vi "Calculate Velocity Setpoints.vi"(0 "Negated":bool, 1 "Front is Back":bool, 3 "Reversed":bool, 4 "Iterations":i32, 5 "Time":u32, 6 "Velocity Data":dbl[](array[numeric]), 7 "Angular Data (Relative)":dbl[](array[numeric]), 9 "Align?":bool, 11 "Enum":enum16{"Vantage", "Mule", "Linda/Sophie"}(ring), 12 "Angle To Get":dbl(slide) scale=0.0..360.0, 13 "IMU Input":dbl, 17 "Commands":cluster{"Time (s)":dbl, T1, bool}[](array[cluster])) -> (2 "Angles PID M":cluster{"Numeric":dbl, "IMU Input":dbl}(graph), 14 "Left Setpoint":dbl, 15 "Wait Time (ms)":dbl, 18 "Finished?":bool, 19 "Right Setpoint":dbl)   [LabVIEW 2019]
uses:
  Bordeaux/Command Stuff/Single Cmd Info.ctl
  <vilib>/picture/picture.llb/imagedata.ctl
  <vilib>/addons/control/pid/pid.llb/PID (DBL).vi
  2020 Robot/Framework/Robot Global Data.vi
  <vilib>/addons/control/pid/NI_PID_pid.lvlib
panel:
  out "Angles PID L/S":cluster{"Numeric":dbl, "IMU Input":dbl}(graph)
  out "Timing Feedback":u32(graph)
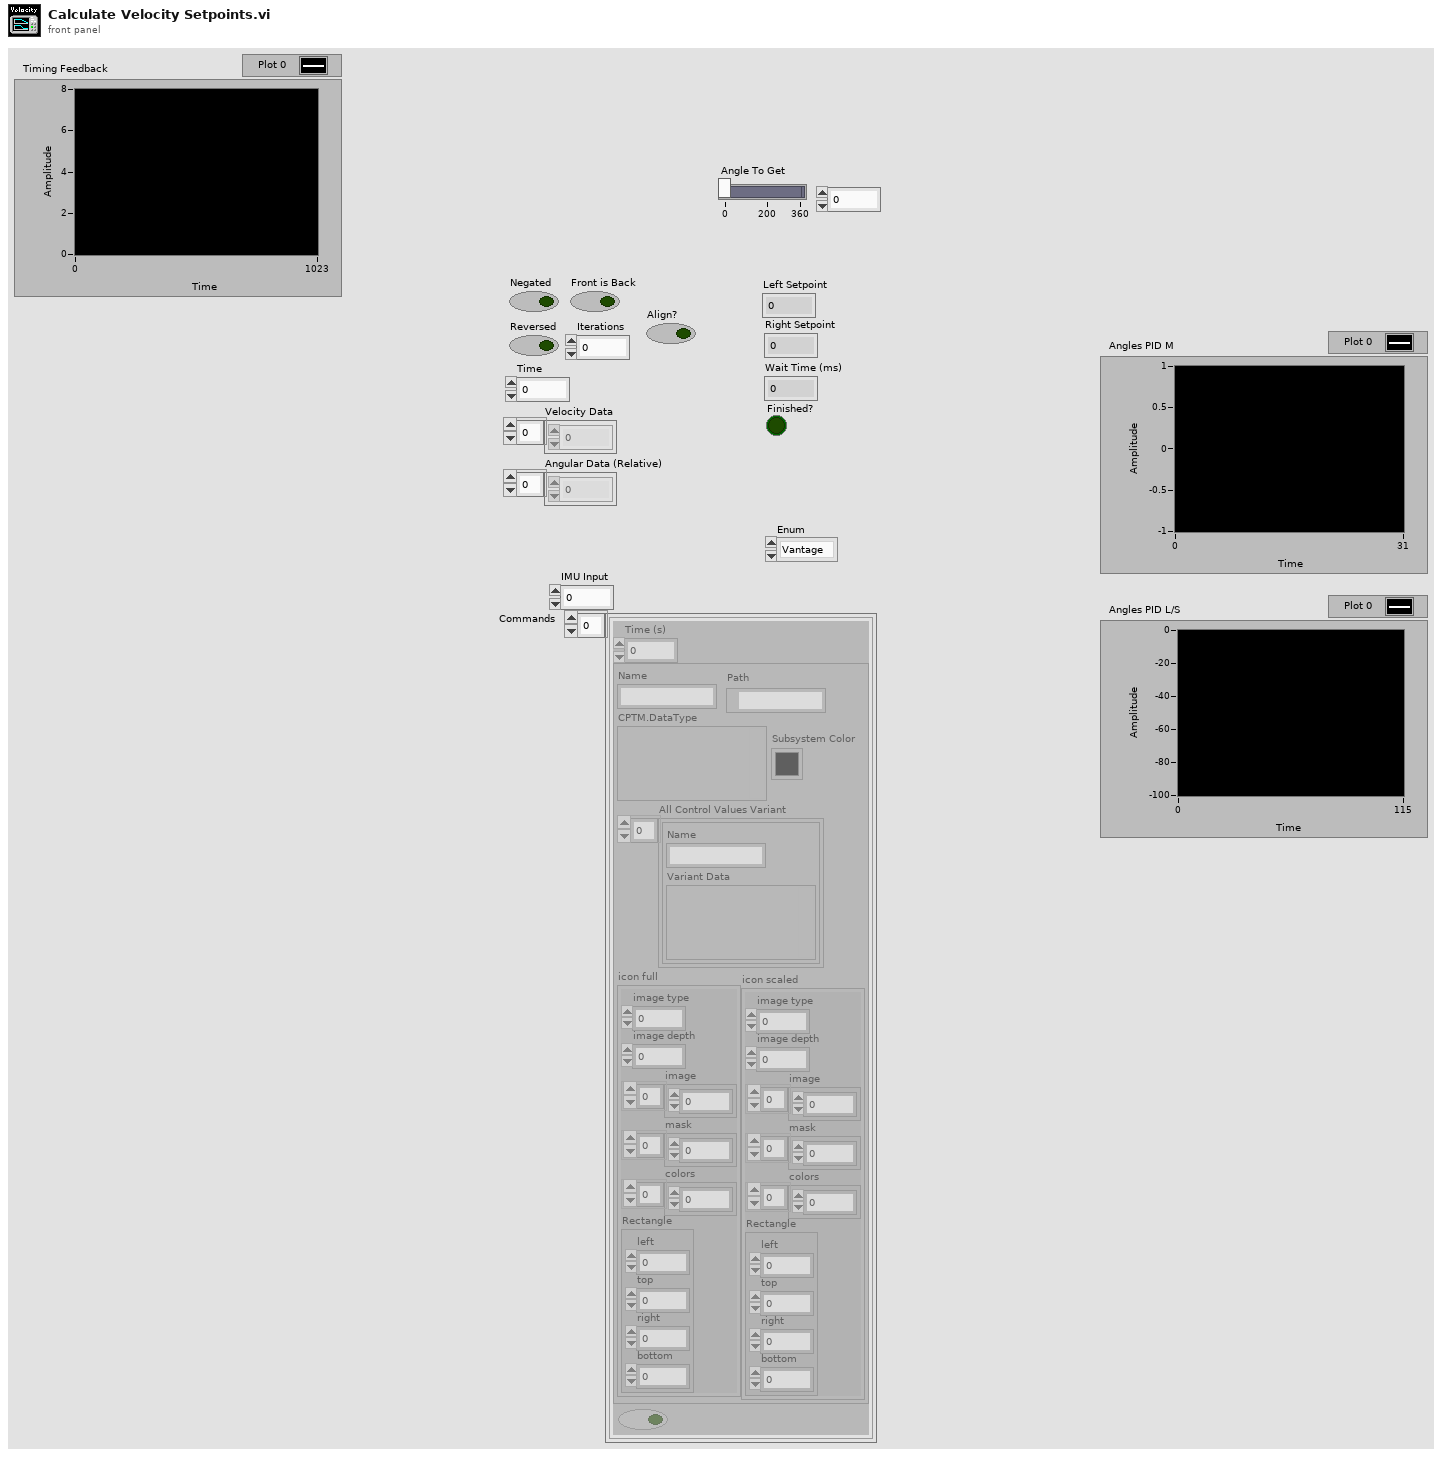
[diagram p1: front panel]
types:
  T1 = typedef "Single Cmd Info.ctl" = cluster{"Name":string, "CPTM.DataType":variant, "All Control Values Variant":cluster{"Name":string, "Variant Data":variant}[], "icon full":T2, "icon scaled":T2, "Path":path, "Subsystem Color":u32}
  T2 = typedef "imagedata.ctl" = cluster{"image type":i32, "image depth":i32, "image":u8[], "mask":u8[], "colors":u32[], "Rectangle":cluster{"left":i16, "top":i16, "right":i16, "bottom":i16}}
  T3 = cluster{"proportional gain (Kc)":dbl, "integral time (Ti, min)":dbl, "derivative time (Td, min)":dbl}
  T4 = enum16{"Vantage", "Mule", "Linda/Sophie", "Rose/Maple"}
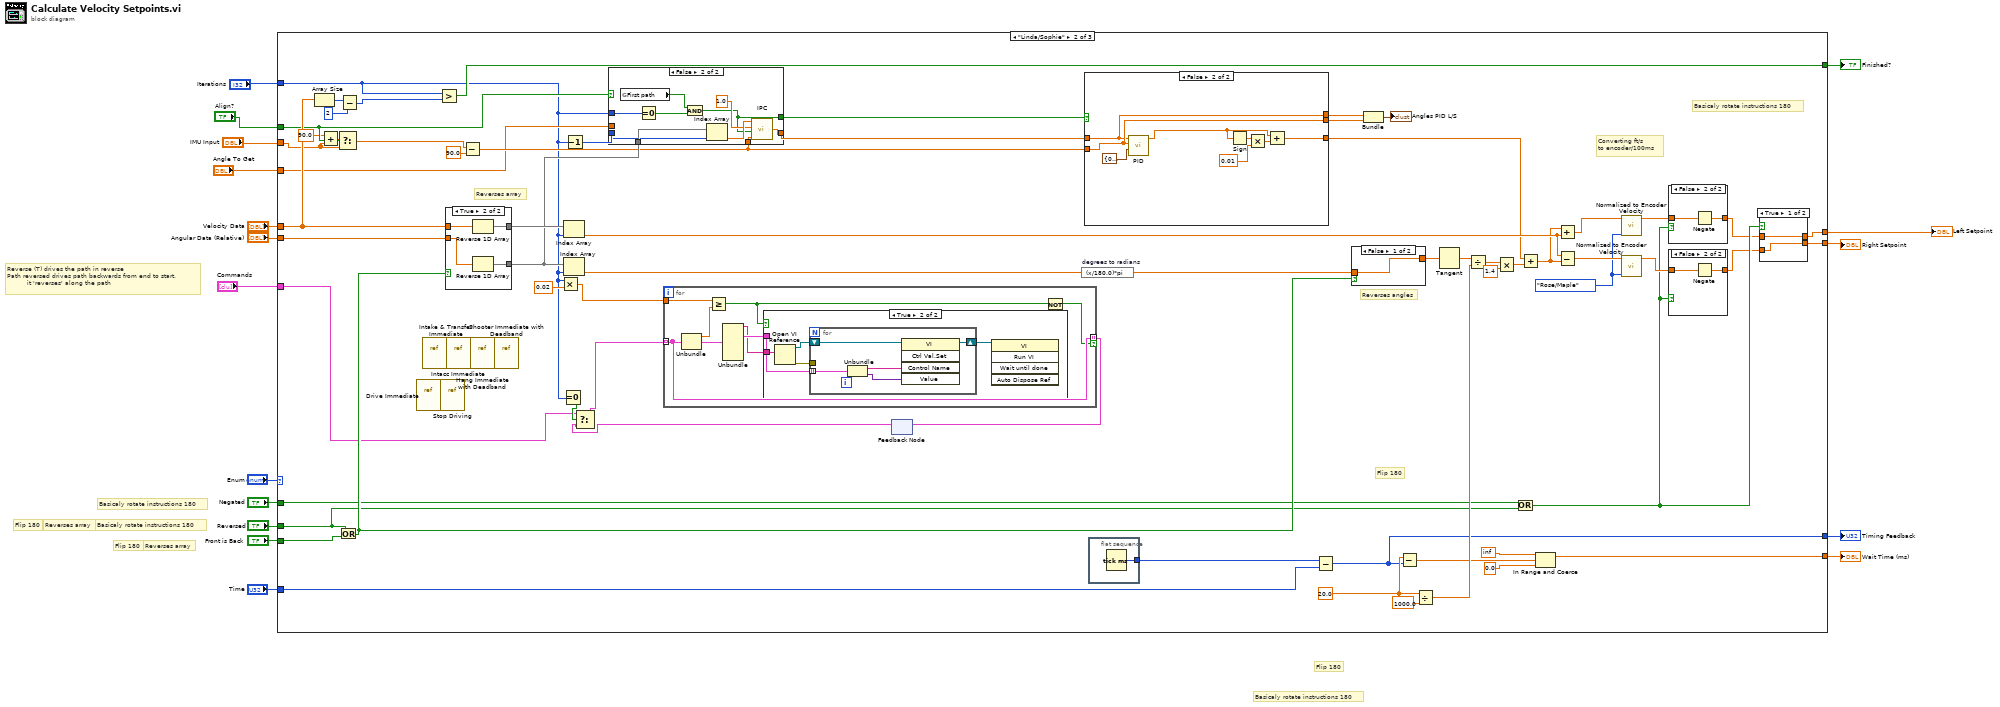
[diagram p0: block diagram]
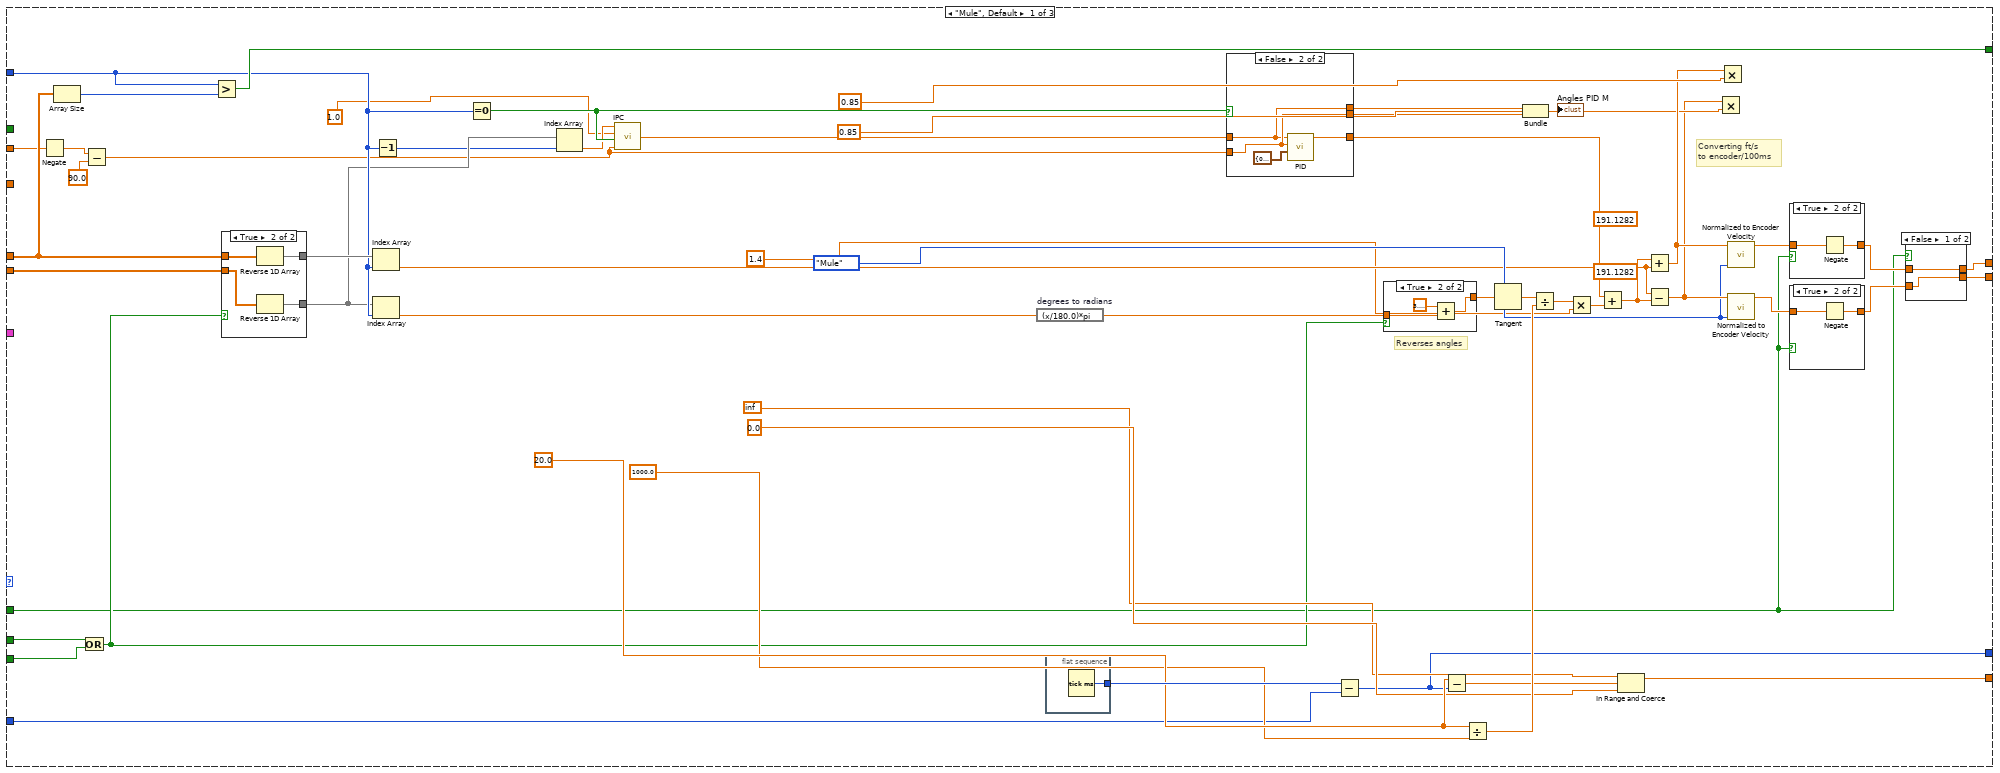
[diagram p2: hidden frame]
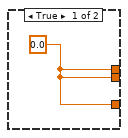
[diagram p4: hidden frame]
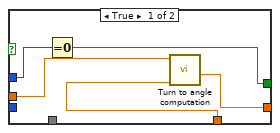
[diagram p10: hidden frame]
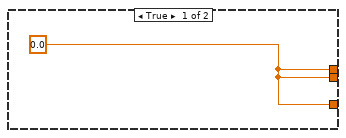
[diagram p12: hidden frame]
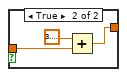
[diagram p14: hidden frame]
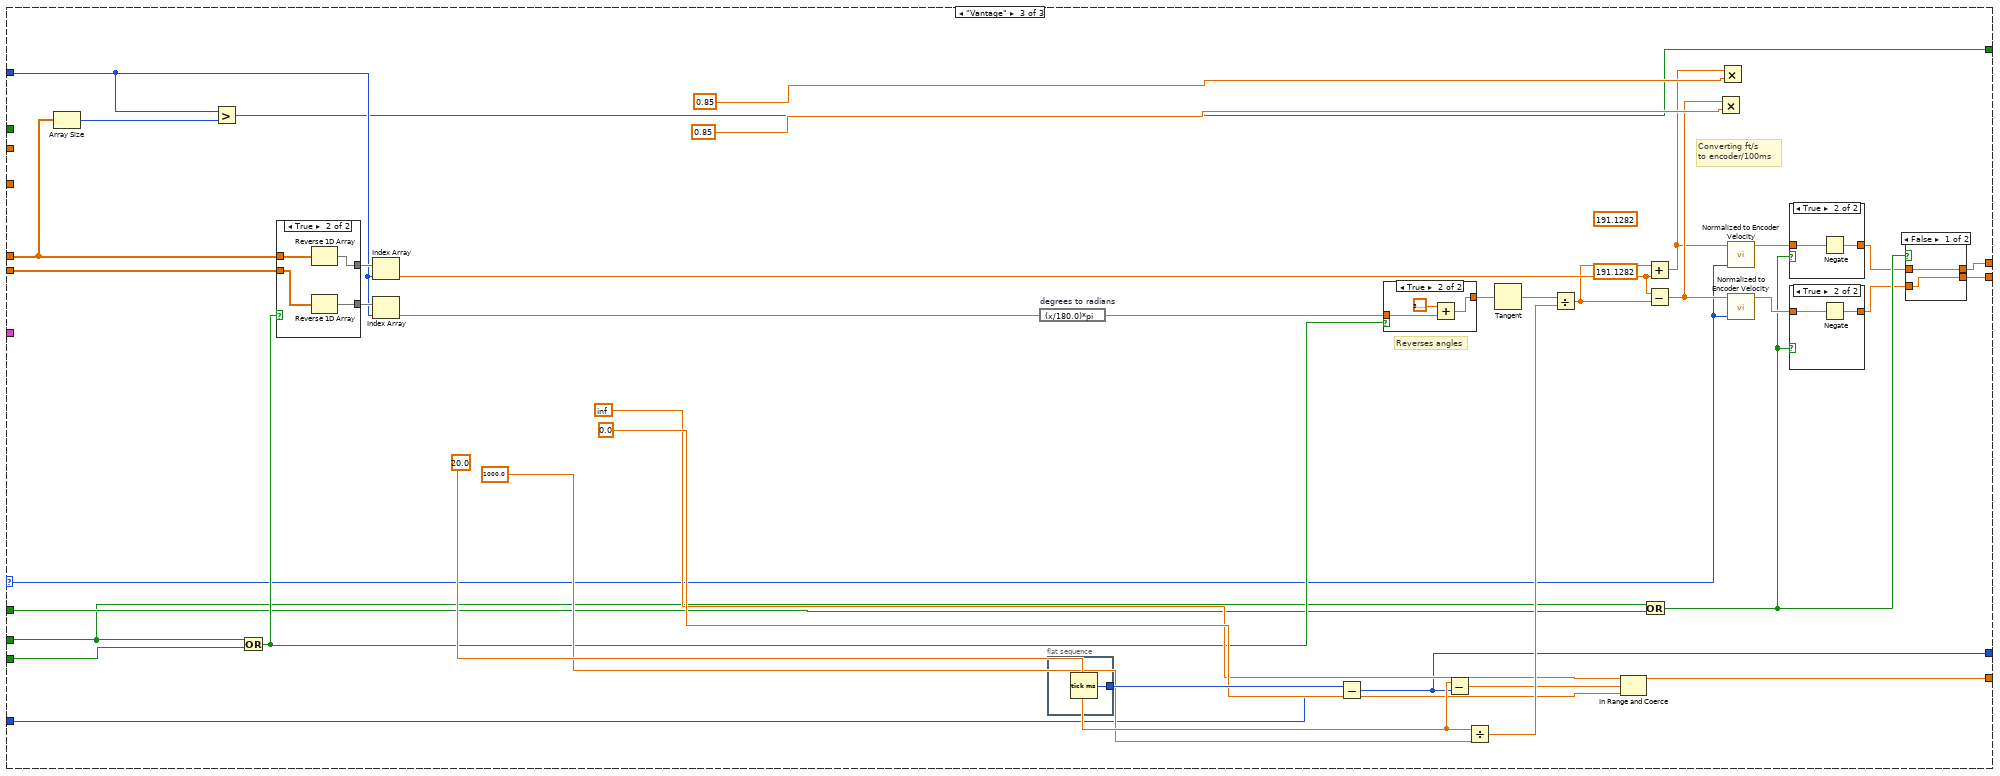
[diagram p17: hidden frame]
diagram:
  # "Reverse (T) drives the path in reverse\nPath reversed drives path backwards from end to start. \n          it 'reverses' along the path"
  # "Basicaly rotate instructions 180"
  # "Basicaly rotate instructions 180"
  # "Flip 180"
  # "Flip 180"
  # "Reverses array"
  # "Reverses array"
  # "Flip 180"
  # "Basicaly rotate instructions 180"
  n1 = case shown="\"Linda/Sophie\"" "Enum" {
    selector: "Enum" -> [_ _ w225]
    tunnel: "Negated" -> [w18 w145 w241]
    tunnel: "Reversed" -> [w55 w144 w240]
    tunnel: "Front is Back" -> [w54 w143 w239]
    tunnel: "Iterations" -> [w27 w104 w238]
    tunnel: "Time" -> [w53 w142 w237]
    tunnel: "Angular Data (Relative)" -> [w52 w141 w236]
    tunnel: "Velocity Data" -> [w51 w140 w235]
    tunnel: [w46 w137 w231] -> w9
    tunnel: [w45 w136 w230] -> w4
    tunnel: [w44 w135 w229] -> w8
    tunnel: [w43 w134 w228] -> w7
    tunnel: [w42 w133 w227] -> w6
    tunnel: "IMU Input" -> [w30 w109 _]
    tunnel: "Align?" -> [_ w112 _]
    tunnel: "Angle To Get" -> [_ w113 _]
    tunnel: "Commands" -> [_ w102 _]
    frame "Mule", Default {
      (unwired) 191.1282 ("y 2")
      (unwired) 191.1282 ("y 2")
      w41 = enum16{"Vantage", "Mule"}."Mule" ("Enum")
      w69 = 20.0 ("x")
      # "Converting ft/s\nto encoder/100ms"
      # "Reverses angles"
      n2 = Negate(x=w30) -> (-x=w29:dbl)
      n3 = Array Size(array=w51) -> (size(s)=w59:i32)
      n4 = Or(x=w55, y=w54) -> (x .or. y?=w58:bool)
      n5 = Subtract(x=w29, y=90.0) -> (x-y=w21:dbl)
      n6 = Greater?(x=w27, y=w59) -> (0:w42:bool)
      n7 = case shown="True" w58 {
        tunnel: [w72 w77] -> w26
        tunnel: [w73 w76] -> w60
        tunnel: w52 -> [w72 w74]
        tunnel: w51 -> [w73 w75]
        frame False {
        }
        frame True {
          n8 = Reverse 1D Array(array=w75) -> (reversed array=w76:dbl[])
          n9 = Reverse 1D Array(array=w74) -> (reversed array=w77:dbl[])
        }
      }
      n10 = Index Array(array=w60, index=w27) -> (element=w40:dbl)
      n11 = Index Array(array=w26, index=w27) -> (element=w38:dbl)
      n12 = Decrement(x=w27) -> (x-1=w25:i32)
      n13 = Equal To 0?(x=w27) -> (x = 0?=w24:bool)
      n14 = Index Array(array=w26, index=w25) -> (element=w23:dbl)
      n15 = call "IPC.vi"("Initilization"=w21, "Reset"=w24, "Multiplier"=1.0, "Value"=w23) -> ("IPCed"=w22:dbl)  [unwired: 2 in]
      n16 = expression code="(x/180.0)*pi" "degrees to radians"(w38) -> (w37:dbl)
      n17 = flat-sequence {
        tunnel: [w78] -> w71
        frame #0 {
          n18 = Tick Count (ms)() -> (millisecond timer value=w78:u32)
        }
      }
      n19 = case shown="False" w24 {
        tunnel: w21 -> [_ w81]
        tunnel: [w79 w82] -> w19
        tunnel: [w79 w80] -> w32
        tunnel: [w79 w81] -> w31
        tunnel: w22 -> [_ w80]
        frame True {
          w79 = 0.0 ("output")
        }
        frame False {
          n20 = call-poly <vilib>:"PID.vi"("PID gains"=T3 {"proportional gain (Kc)"=0.2, "integral time (Ti, min)"=0.4, "derivative time (Td, min)"=0.0006} ("PID gains M"), "process variable"=w81, "setpoint"=w80) -> ("output"=w82:dbl)  [unwired: 7 in, 1 out]
        }
      }
      n21 = Subtract(x=w71, y=w53) -> (x-y=w43:u32)
      n22 = case shown="True" w58 {
        tunnel: w37 -> [w88 w91]
        tunnel: [w88 w90] -> w61
        frame False {
        }
        frame True {
          n23 = Add(x=3.141592653589793, y=w91) -> (x+y=w90:dbl)
        }
      }
      n24 = Subtract(x=w69, y=w43) -> (x-y=w65:dbl)
      n25 = Divide(x=w69, y=1000.0) -> (x/y=w67:dbl)
      n26 = Tangent(1:w61) -> (0:w70:dbl)
      n27 = Bundle("IPCed"=w32, "output"=w31) -> (→"Angles PID M":cluster{"IPCed":dbl, "output":dbl})  [unwired: 1 in]
      n28 = Divide(x=w70, y=w67) -> (x/y=w39:dbl)
      n29 = Multiply(x=w39, y=1.4) -> (x*y=w35:dbl)
      n30 = Add(x=w19, y=w35) -> (x+y=w34:dbl)
      n31 = In Range and Coerce(upper limit=inf, x=w65, lower limit=0.0) -> (coerced(x)=w44:dbl)  [unwired: 1 out]
      n32 = Add(x=w34, y=w40) -> (x+y=w49:dbl)
      n33 = Subtract(x=w40, y=w34) -> (x-y=w47:dbl)
      n34 = Multiply(x=w47, y=0.85) -> ()  [unwired: 1 out]
      n35 = Multiply(x=w49, y=0.85) -> ()  [unwired: 1 out]
      n36 = call "Normalized to Encoder Velocity.vi"("Enum"=w41, "ft/s"=w49) -> ("Output"=w63:dbl)  [unwired: 9 in]
      n37 = call "Normalized to Encoder Velocity.vi"("Enum"=w41, "ft/s"=w47) -> ("Output"=w62:dbl)  [unwired: 9 in]
      n38 = case shown="True" w18 {
        tunnel: w63 -> [w95 w97]
        tunnel: [w95 w96] -> w57
        frame False {
        }
        frame True {
          n39 = Negate(x=w97) -> (-x=w96:dbl)
        }
      }
      n40 = case shown="True" w18 {
        tunnel: [w92 w94] -> w56
        tunnel: w62 -> [w92 w93]
        frame False {
        }
        frame True {
          n41 = Negate(x=w93) -> (-x=w94:dbl)
        }
      }
      n42 = case shown="False" w18 {
        tunnel: w56 -> [w85 w86]
        tunnel: w57 -> [w84 w87]
        tunnel: [w85 w87] -> w46
        tunnel: [w84 w86] -> w45
        frame False {
        }
        frame True {
        }
      }
    }
    frame "Linda/Sophie" {
      w98 = T4."Rose/Maple" ("Enum")
      w159 = 20.0 ("x")
      # "Basicaly rotate instructions 180"
      # "Flip 180"
      # "Reverses array"
      # "Converting ft/s\nto encoder/100ms"
      # "Reverses angles"
      n43 = Array Size(array=w140) -> (size(s)=w116:i32)
      n44 = Add(x=90.0, y=w109) -> (x+y=w110:dbl)
      n45 = Select(t=w110, s=w112, f=w109) -> (s? t:f=w107:dbl)
      n46 = Or(x=w144, y=w143) -> (x .or. y?=w149:bool)
      n47 = Subtract(x=w116, y=2) -> (x-y=w115:i32)
      n48 = vi-ref "Drive Immediate.vi"() -> ()  [unwired: 1 out]
      n49 = vi-ref "Intake & Transfer Immediate.vi"() -> ()  [unwired: 1 out]
      n50 = Greater?(x=w104, y=w115) -> (0:w133:bool)
      n51 = vi-ref "Stop Driving.vi"() -> ()  [unwired: 1 out]
      n52 = case shown="True" w149 {
        tunnel: [w195 w200] -> w122
        tunnel: [w196 w199] -> w150
        tunnel: w141 -> [w195 w197]
        tunnel: w140 -> [w196 w198]
        frame False {
        }
        frame True {
          n53 = Reverse 1D Array(array=w198) -> (reversed array=w199:dbl[])
          n54 = Reverse 1D Array(array=w197) -> (reversed array=w200:dbl[])
        }
      }
      n55 = vi-ref "Intacc Immediate.vi"() -> ()  [unwired: 1 out]
      n56 = Subtract(x=w107, y=90.0) -> (x-y=w118:dbl)
      n57 = vi-ref "Hang Immediate with Deadband.vi"() -> ()  [unwired: 1 out]
      n58 = vi-ref "Shooter Immediate with Deadband.vi"() -> ()  [unwired: 1 out]
      n59 = Multiply(x=w104, y=0.02 ("x")) -> (x*y=w105:dbl)
      n60 = Equal To 0?(x=w104) -> (x = 0?=w103:bool)
      n61 = Index Array(array=w150, index=w104) -> (element=w132:dbl)
      n62 = Index Array(array=w122, index=w104) -> (element=w130:dbl)
      n63 = Decrement(x=w104) -> (x-1=w121:i32)
      n64 = case shown="False" w112 {
        tunnel: w104 -> [w181 w194]
        tunnel: w122 -> [_ w193]
        tunnel: w121 -> [_ w192]
        tunnel: [w180 w186] -> w120
        tunnel: [w182 w190] -> w119
        tunnel: w118 -> [w184 w189]
        tunnel: w113 -> [w183 _]
        frame True {
          n65 = Equal To 0?(x=w181) -> (x = 0?=w180:bool)
          n66 = call "Turn to angle computation.vi"("Current Angle"=w184, "Angle To Get"=w183) -> ("New Angle to get"=w182:dbl)  [unwired: 9 in]
        }
        frame False {
          n67 = global read "Robot Global Data.vi" "First path"() -> (w185:bool)
          n68 = Equal To 0?(x=w194) -> (x = 0?=w187:bool)
          n69 = And(x=w185, y=w187) -> (x .and. y?=w186:bool)
          n70 = Index Array(array=w193, index=w192) -> (element=w191:dbl)
          n71 = call "IPC.vi"("Initilization"=w189, "Reset"=w186, "Multiplier"=1.0, "Value"=w191) -> ("IPCed"=w190:dbl)  [unwired: 2 in]
        }
      }
      n72 = feedback #1() -> (w99:cluster{"Time (s)":dbl, T1, bool}[])  [unwired: 1 in]
      n73 = Select(t=w102, s=w103, f=w99) -> (s? t:f=w101:cluster{"Time (s)":dbl, T1, bool}[])
      n74 = for {
        tunnel: w101 -> [w169] mode=indexing
        tunnel: w105 -> [w167]
        tunnel: [w169] -> w100 mode=indexing if=w164
        n75 = Unbundle(w169) -> ("Time (s)"=w168:dbl, w166:T1)  [unwired: 1 out]
        n76 = Greater Or Equal?(x=w167, y=w168) -> (x >= y?=w163:bool)
        n77 = Unbundle(w166) -> ("Name"=w162:string, "All Control Values Variant"=w165:cluster{"Name":string, "Variant Data":variant}[])  [unwired: 5 out]
        n78 = case shown="True" w163 {
          tunnel: w162 -> [_ w174]
          tunnel: w165 -> [_ w173]
          frame False {
          }
          frame True {
            n79 = Open VI Reference(vi path=w174) -> (vi reference=w172:refnum<vi>, error out=w170:errorcluster)  [unwired: 5 in]
            n80 = for {
              tunnel: w173 -> [w179] mode=indexing
              shift-right: [w176] -> w171
              shift-left: w172 -> [w175]
              tunnel: w170 -> [_]
              n81 = Unbundle(w179) -> ("Name"=w178:string, "Variant Data"=w177:variant)
              n82 = invoke class="VI" method="Ctrl Val.Set"(reference=w175, "Control Name"=w178, "Value"=w177) -> (reference out=w176:refnum<vi>)  [unwired: 2 in, 4 out]
            }
            n83 = invoke class="VI" method="Run VI"(reference=w171) -> ()  [unwired: 4 in, 5 out]
          }
        }
        n84 = Not(x=w163) -> (.not. x?=w164:bool)
      }
      n85 = feedback-in #1(w100) -> ()
      n86 = expression code="(x/180.0)*pi" "degrees to radians"(w130) -> (w129:dbl)
      n87 = case shown="False" w120 {
        tunnel: w118 -> [_ w210]
        tunnel: [w202 w206] -> w117
        tunnel: [w202 w209] -> w124
        tunnel: [w202 w210] -> w123
        tunnel: w119 -> [_ w209]
        frame True {
          w202 = 0.0 ("output")
        }
        frame False {
          n88 = call-poly <vilib>:"PID.vi"("PID gains"=T3 {"proportional gain (Kc)"=0.08, "integral time (Ti, min)"=0.0, "derivative time (Td, min)"=0.001} ("PID gains L/S 2"), "process variable"=w210, "setpoint"=w209) -> ("output"=w205:dbl)  [unwired: 7 in, 1 out]
          n89 = Sign(1:w205) -> (0:w208:dbl)
          n90 = Multiply(x=w208, y=0.01 ("f")) -> (x*y=w207:dbl)
          n91 = Add(x=w205, y=w207) -> (x+y=w206:dbl)
        }
      }
      n92 = flat-sequence {
        tunnel: [w201] -> w161
        frame #0 {
          n93 = Tick Count (ms)() -> (millisecond timer value=w201:u32)
        }
      }
      n94 = Subtract(x=w161, y=w142) -> (x-y=w134:u32)
      n95 = case shown="False" w149 {
        tunnel: w129 -> [w215 w218]
        tunnel: [w215 w217] -> w151
        frame False {
        }
        frame True {
          n96 = Add(x=3.141592653589793, y=w218) -> (x+y=w217:dbl)
        }
      }
      n97 = Bundle("IPCed"=w124, "output"=w123) -> (→"Angles PID L/S":cluster{"IPCed":dbl, "output":dbl})  [unwired: 1 in]
      n98 = Subtract(x=w159, y=w134) -> (x-y=w155:dbl)
      n99 = Divide(x=w159, y=1000.0) -> (x/y=w157:dbl)
      n100 = Tangent(1:w151) -> (0:w160:dbl)
      n101 = Divide(x=w160, y=w157) -> (x/y=w131:dbl)
      n102 = Multiply(x=w131, y=1.4) -> (x*y=w127:dbl)
      n103 = Or(x=w145, y=w144) -> (x .or. y?=w148:bool)
      n104 = Add(x=w117, y=w127) -> (x+y=w126:dbl)
      n105 = In Range and Coerce(upper limit=inf, x=w155, lower limit=0.0) -> (coerced(x)=w135:dbl)  [unwired: 1 out]
      n106 = Add(x=w126, y=w132) -> (x+y=w139:dbl)
      n107 = Subtract(x=w132, y=w126) -> (x-y=w138:dbl)
      n108 = call "Normalized to Encoder Velocity.vi"("Enum"=w98, "ft/s"=w139) -> ("Output"=w153:dbl)  [unwired: 9 in]
      n109 = call "Normalized to Encoder Velocity.vi"("Enum"=w98, "ft/s"=w138) -> ("Output"=w152:dbl)  [unwired: 9 in]
      n110 = case shown="False" w148 {
        tunnel: w153 -> [w222 w224]
        tunnel: [w222 w223] -> w147
        frame True {
        }
        frame False {
          n111 = Negate(x=w224) -> (-x=w223:dbl)
        }
      }
      n112 = case shown="False" w148 {
        tunnel: [w219 w221] -> w146
        tunnel: w152 -> [w219 w220]
        frame True {
        }
        frame False {
          n113 = Negate(x=w220) -> (-x=w221:dbl)
        }
      }
      n114 = case shown="True" w148 {
        tunnel: w146 -> [w212 w213]
        tunnel: w147 -> [w211 w214]
        tunnel: [w212 w214] -> w137
        tunnel: [w211 w213] -> w136
        frame True {
        }
        frame False {
        }
      }
    }
    frame "Vantage" {
      (unwired) 191.1282 ("y 2")
      (unwired) 191.1282 ("y 2")
      w259 = 20.0 ("x")
      # "Converting ft/s\nto encoder/100ms"
      # "Reverses angles"
      n115 = Array Size(array=w235) -> (size(s)=w246:i32)
      n116 = Greater?(x=w238, y=w246) -> (0:w227:bool)
      n117 = Or(x=w240, y=w239) -> (x .or. y?=w245:bool)
      n118 = case shown="True" w245 {
        tunnel: [w264 w269] -> w249
        tunnel: [w265 w268] -> w248
        tunnel: w236 -> [w264 w266]
        tunnel: w235 -> [w265 w267]
        frame False {
        }
        frame True {
          n119 = Reverse 1D Array(array=w267) -> (reversed array=w268:dbl[])
          n120 = Reverse 1D Array(array=w266) -> (reversed array=w269:dbl[])
        }
      }
      n121 = Index Array(array=w248, index=w238) -> (element=w262:dbl)
      n122 = Index Array(array=w249, index=w238) -> (element=w247:dbl)
      n123 = expression code="(x/180.0)*pi" "degrees to radians"(w247) -> (w251:dbl)
      n124 = flat-sequence {
        tunnel: [w270] -> w263
        frame #0 {
          n125 = Tick Count (ms)() -> (millisecond timer value=w270:u32)
        }
      }
      n126 = Subtract(x=w263, y=w237) -> (x-y=w228:u32)
      n127 = case shown="True" w245 {
        tunnel: w251 -> [w275 w278]
        tunnel: [w275 w277] -> w250
        frame False {
        }
        frame True {
          n128 = Add(x=3.141592653589793, y=w278) -> (x+y=w277:dbl)
        }
      }
      n129 = Subtract(x=w259, y=w228) -> (x-y=w255:dbl)
      n130 = Divide(x=w259, y=1000.0) -> (x/y=w257:dbl)
      n131 = Tangent(1:w250) -> (0:w261:dbl)
      n132 = Divide(x=w261, y=w257) -> (x/y=w260:dbl)
      n133 = In Range and Coerce(upper limit=inf, x=w255, lower limit=0.0) -> (coerced(x)=w229:dbl)  [unwired: 1 out]
      n134 = Or(x=w240, y=w241) -> (x .or. y?=w244:bool)
      n135 = Add(x=w260, y=w262) -> (x+y=w226:dbl)
      n136 = Subtract(x=w262, y=w260) -> (x-y=w232:dbl)
      n137 = Multiply(x=w232, y=0.85) -> ()  [unwired: 1 out]
      n138 = Multiply(x=w226, y=0.85) -> ()  [unwired: 1 out]
      n139 = call "Normalized to Encoder Velocity.vi"("Enum"=w225, "ft/s"=w226) -> ("Output"=w253:dbl)  [unwired: 9 in]
      n140 = call "Normalized to Encoder Velocity.vi"("Enum"=w225, "ft/s"=w232) -> ("Output"=w252:dbl)  [unwired: 9 in]
      n141 = case shown="True" w244 {
        tunnel: w253 -> [w282 w284]
        tunnel: [w282 w283] -> w243
        frame False {
        }
        frame True {
          n142 = Negate(x=w284) -> (-x=w283:dbl)
        }
      }
      n143 = case shown="True" w244 {
        tunnel: [w279 w281] -> w242
        tunnel: w252 -> [w279 w280]
        frame False {
        }
        frame True {
          n144 = Negate(x=w280) -> (-x=w281:dbl)
        }
      }
      n145 = case shown="False" w244 {
        tunnel: w242 -> [w272 w273]
        tunnel: w243 -> [w271 w274]
        tunnel: [w272 w274] -> w231
        tunnel: [w271 w273] -> w230
        frame False {
        }
        frame True {
        }
      }
    }
  }
  "Left Setpoint" <- w4
  "Right Setpoint" <- w9
  "Wait Time (ms)" <- w8
  "Timing Feedback" <- w7
  "Finished?" <- w6
